vi "Read MaxElapsedTime.vi"(8 "error in (no error)":errorcluster, 11 "Watchdog in":refnum<class "Watchdog.lvclass">) -> (0 "error out":errorcluster, 2 "MaxElapsedTime":u32, 3 "Watchdog out":refnum<class "Watchdog.lvclass">)   [LabVIEW 2017, in "Watchdog.lvclass"]
uses:
  <vilib>/NI/Software Watchdog/Watchdog/Watchdog.lvclass
  <vilib>/NI/Software Watchdog/Watchdog/Watchdog.lvclass/Watchdog.ctl
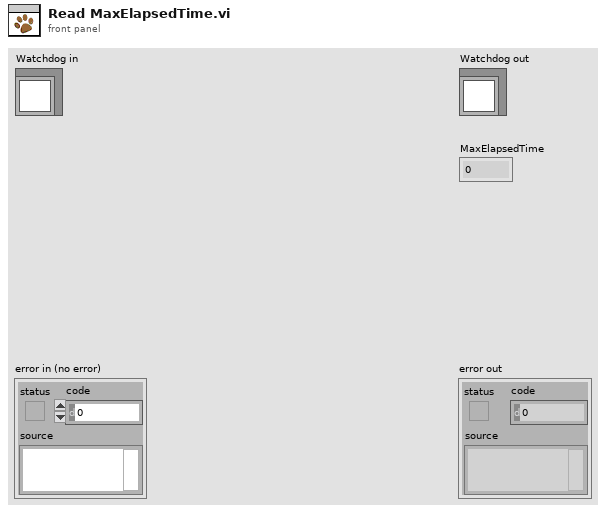
[diagram p1: front panel]
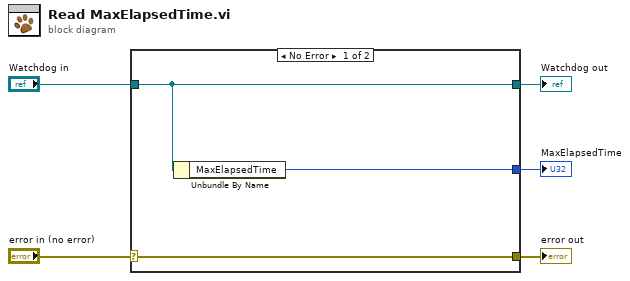
[diagram p0: block diagram]
diagram:
  n1 = case shown="No Error" "error in (no error)" {
    selector: "error in (no error)" -> [w8 w9]
    tunnel: [w8 w9] -> w4
    tunnel: [w7 w10] -> w2
    tunnel: "Watchdog in" -> [w7 w10]
    tunnel: [w6 _] -> w1
    frame No Error {
      n2 = Unbundle By Name(w7) -> ("MaxElapsedTime"=w6:u32)
    }
    frame Error {
    }
  }
  "error out" <- w4
  "Watchdog out" <- w2
  "MaxElapsedTime" <- w1
